vi "Wrap Data.vi"(7 "Start Time":timestamp, 8 "error in (no error)":errorcluster, 9 "Data in":refnum<class "Data.lvclass">, 10 "Actor in":refnum<class "Actor.lvclass">, 11 "Timed Msg":refnum<class "Timed Msg.lvclass">) -> (0 "error out":errorcluster, 1 "Data out":refnum<class "Data.lvclass">, 2 "Actor out":refnum<class "Actor.lvclass">)   [LabVIEW 2020, in "Publisher.lvlib" / "Timed Msg.lvclass"]
doc: "The Wrap Data VI allows the Actor and/or message to interact with the data before it is sent or published.\n\nThis implementation adds timed info if the Data is part of the Timed Data hierarchy."
uses:
  Timed Msg.lvclass
  PPL/HDH.Actor Framework.Core.Actor.lvlibp/1abvi3w/vi.lib/ActorFramework/Actor/Actor.lvclass
  PPL/HDH.Data.Generic.lvlibp/Data.lvclass
  Data/Timed Data/Timed Data.lvclass
  C:/Current projects/WS/PPL/HDH.Data.Generic.lvlibp/Data.lvclass
  Data/Timed Data/Timed Data.lvclass/Timed Data.ctl
  Response Msg/Response Msg.lvclass
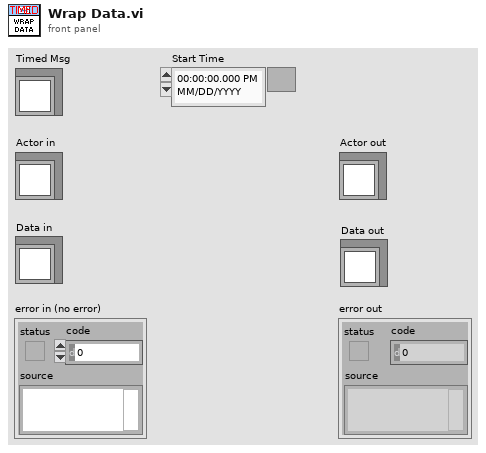
[diagram p1: front panel]
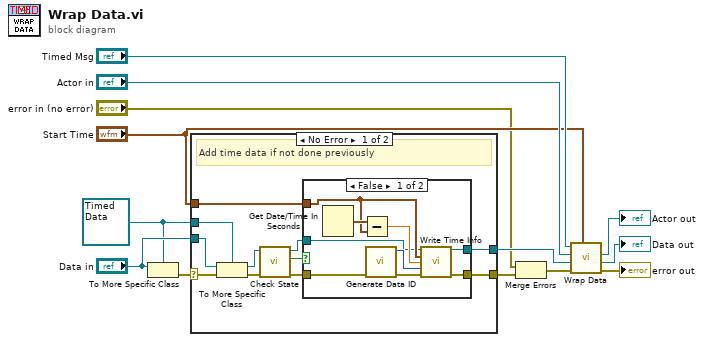
[diagram p0: block diagram]
diagram:
  w3 = refnum<class "Timed Data.lvclass"> refnum ("Publisher.lvlib:Timed Data.lvclass")
  n1 = To More Specific Class(target class=w3, reference="Data in") -> (error out=w8:errorcluster)  [unwired: 1 in, 1 out]
  n2 = case shown="No Error" w8 {
    selector: w8 -> [w24 _]
    tunnel: [w20 w36] -> w7
    tunnel: "Data in" -> [w23 w36]
    tunnel: "Start Time" -> [w21 _]
    tunnel: [w19 _] -> w4
    tunnel: w3 -> [w22 _]
    frame No Error {
      # "Add time data if not done previously"
      n3 = To More Specific Class(target class=w22, reference=w23, error in=w24) -> (specific class reference=w18:refnum<class "Timed Data.lvclass">, error out=w16:errorcluster)
      n4 = call "Check State.vi"("error in (no error)"=w16, "Timed Data in"=w18) -> ("error out"=w15:errorcluster, "Previously Populated?"=w14:bool, "Timed Data out"=w17:refnum<class "Timed Data.lvclass">)  [unwired: 7 in]
      n5 = case shown="False" w14 {
        tunnel: w21 -> [w32 _]
        tunnel: [w31 w35] -> w20
        tunnel: [w30 w34] -> w19
        tunnel: w17 -> [w26 w35]
        tunnel: w15 -> [w25 w34]
        frame False {
          n6 = Get Date/Time In Seconds() -> (seconds since 1Jan1904=w33:timestamp)
          n7 = Subtract(x=w33, y=w32) -> (x-y=w27:dbl)
          n8 = call "Generate Data ID.vi"("error in (no error)"=w25) -> ("error out"=w29:errorcluster, "Data ID"=w28:u32)  [unwired: 9 in]
          n9 = call "Write Time Info.vi"("Request Data in"=w26, "Start TIme"=w32, "Duration(s)"=w27, "Data ID"=w28, "error in (no error)"=w29) -> ("Request Data out"=w31:refnum<class "Timed Data.lvclass">, "error out"=w30:errorcluster)  [unwired: 9 in]
        }
        frame True {
        }
      }
    }
    frame Error {
      # "Not a Timed Data class"
    }
  }
  n10 = Merge Errors("error in (no error)", w4) -> (w2:errorcluster)
  n11 = call-parent "Wrap Data.vi"("Start Time"="Start Time", "error in (no error)"=w2, "Data in"=w7, "Actor in"="Actor in", "Response Msg"="Timed Msg") -> ("error out"=→"error out":errorcluster, "Data out"=→"Data out":refnum<class "Data.lvclass">, "Actor out"=→"Actor out":refnum<class "Actor.lvclass">)  [unwired: 4 in]
